vi "Brewer Palette Dialog v2.vi"() -> (0 "OK?":bool, 1 "Cancelled?":bool, 2 "Interpolate?":bool, 3 "Selected Palette Colors":u32[](array[colorbox]), 5 "Palette Name (# Colors)":string)   [LabVIEW 2021]
doc: "The Palette Colors array returned was chosen by the user while it was displayed vertically.\nIn other words, the top color is in fact color index 0, while the bottom color is in fact the last color in the array.\nTo use this array for a color ramp (or color scale), this array will need to be inverted to obtain the same visual effect."
panel:
  in  "Show Tip Strip":bool
  out "Max  # Colors":i32=3 min=3 max=12 step=1
  in  "About":bool
  in  "Interpolate":bool
  in  "Flip Order":bool
  out "Color Ramp":dbl(ramp)
  in  "Palette List":string(combo)
  in  "Cancel":bool
  in  "OK":bool
  out "Palette Colors":u32[](array[colorbox])
  out "# Palettes":i32=3 min=3 max=12 step=1
  in  "Category":T1(ring)
  in  "photocopy safe":bool
  in  "printer friendly":bool
  in  "colorblind safe":bool
  in  "# Colors":i32=3 min=3 max=15 step=1
  in  "Background":u32(colorbox)=16777226
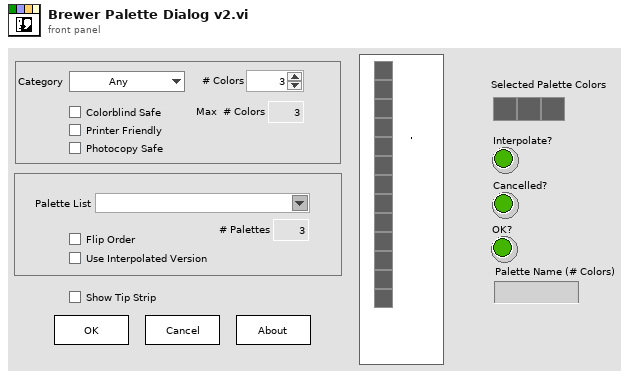
[diagram p1: front panel]
types:
  T1 = enum16{"Any", "Sequential", "Diverging", "Qualitative"}
  T2 = cluster{"Category":enum16{"Any", "Sequential", "Diverging", "Qualitative"}, "photocopy safe":bool, "printer friendly":bool, "colorblind safe":bool, "# Colors":i32, "Flip Order":bool}
  T3 = typedef "Color Brewer Palette.ctl" = cluster{"Color Array":u32[], "Palette Name":string, "Number of Colors":i32, "Palette Category":string, "Color Blind Safe":bool, "Printer Friendly":bool, "Photocopy Safe":bool}
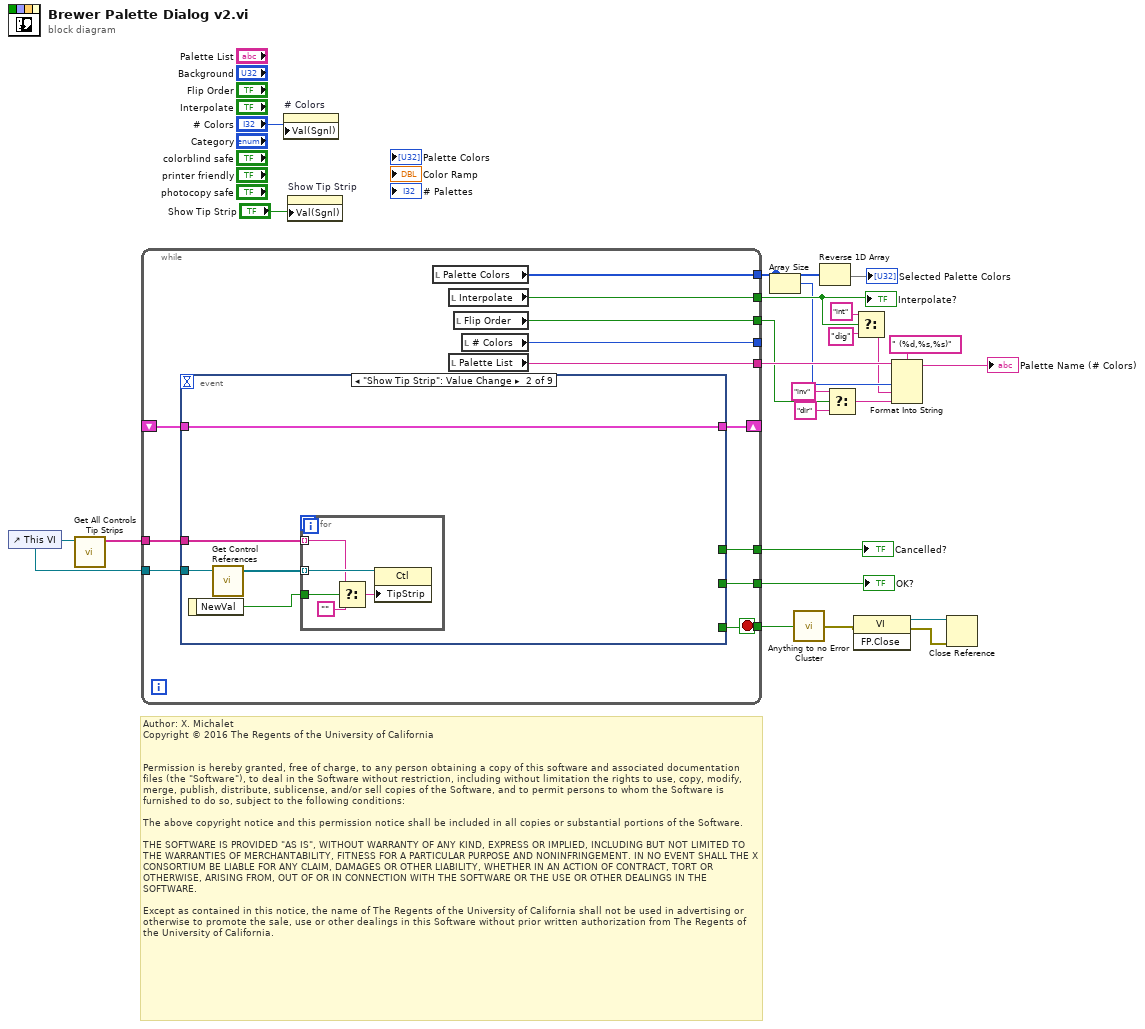
[diagram p0: block diagram]
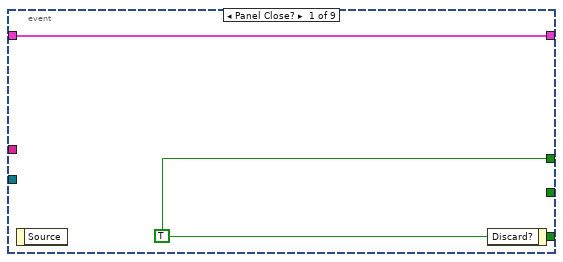
[diagram p2: hidden frame]
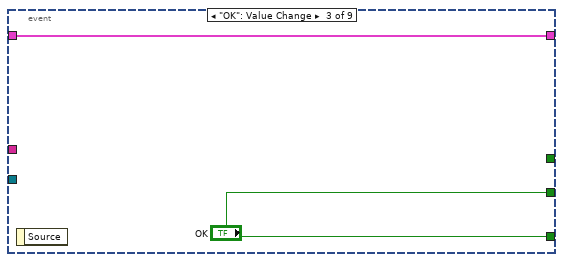
[diagram p3: hidden frame]
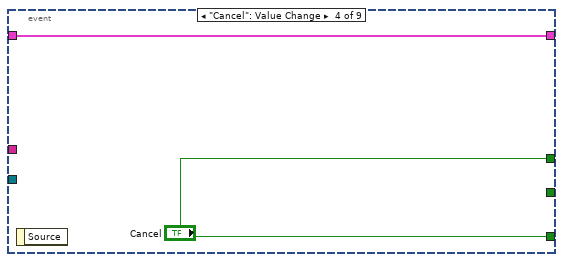
[diagram p4: hidden frame]
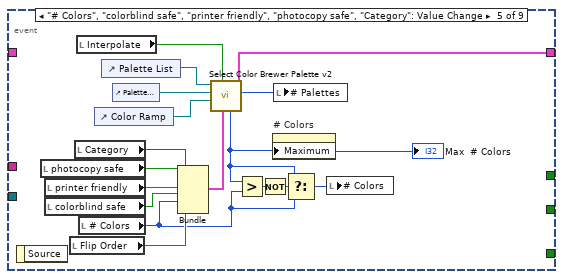
[diagram p5: hidden frame]
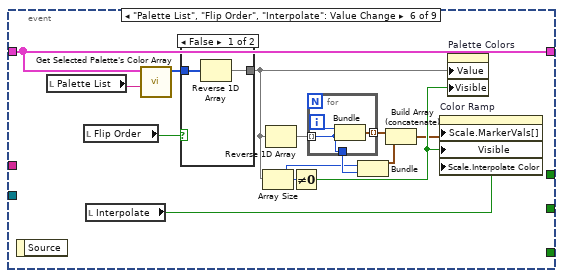
[diagram p6: hidden frame]
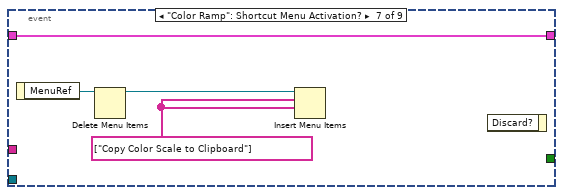
[diagram p8: hidden frame]
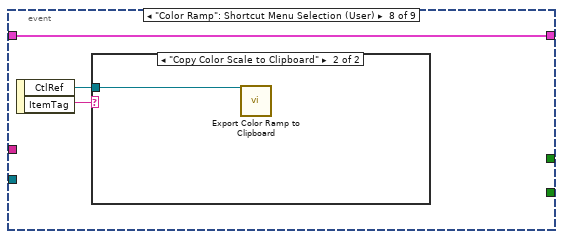
[diagram p9: hidden frame]
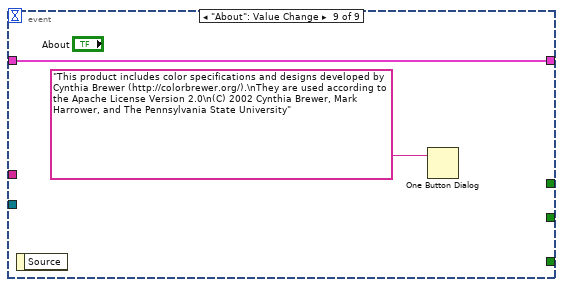
[diagram p11: hidden frame]
diagram:
  # "Author: X. Michalet\nCopyright © 2016 The Regents of the University of California\n \n\nPermission is hereby granted, free of charge, to any person obtaining a copy of this software and associated documentation files (the \"Software\"), to deal in the Software without restriction, including without limitation the rights to use, copy, modify, merge, publish, distribute, sublicense, and/or sell copies of the Software, and to permit persons to whom the Software is furnished to do so, subject to the following conditions:\n\nThe above copyright notice and this permission notice shall be included in all copies or substantial portions of the Software.\n\nTHE SOFTWARE IS PROVIDED \"AS IS\", WITHOUT WARRANTY OF ANY KIND, EXPRESS OR IMPLIED, INCLUDING BUT NOT LIMITED TO THE WARRANTIES OF MERCHANTABILITY, FITNESS FOR A PARTICULAR PURPOSE AND NONINFRINGEMENT. IN NO EVENT SHALL THE X CONSORTIUM BE LIABLE FOR ANY CLAIM, DAMAGES OR OTHER LIABILITY, WHETHER IN AN ACTION OF CONTRACT, TORT OR OTHERWISE, ARISING FROM, OUT OF OR IN CONNECTION WITH THE SOFTWARE OR THE USE OR OTHER DEALINGS IN THE SOFTWARE.\n\nExcept as contained in this notice, the name of The Regents of the University of California shall not be used in advertising or otherwise to promote the sale, use or other dealings in this Software without prior written authorization from The Regents of the University of California."
  n1 = control-ref of="This VI"() -> (w4:refnum<vi>)
  n2 = call "Get All Controls Tip Strips.vi"("VI Ref"=w4) -> ("Controls Tip Strips"=w6:string[])  [unwired: 9 in, 1 out]
  n3 = while {
    shift-right: [w36] -> _
    shift-left: _ -> [w35]
    tunnel: [w34] -> w24
    tunnel: [w33] -> w23
    tunnel: [w32] -> w20
    tunnel: [w31] -> _
    tunnel: [w30] -> w17
    tunnel: [w29] -> w15
    tunnel: [w28] -> w16
    tunnel: w4 -> [w27]
    tunnel: w6 -> [w26]
    tunnel: [w25] -> w2
    stop <- w25 stop-if-true
    n4 = event shown="[1] \"Show Tip Strip\": Value Change" {
      selector: _ -> [_ _ _ _ _ _ _ _ _]
      dyn-events: _ -> [_ _ _ _ _ _ _ _ _]
      timeout: _ -> [_ _ _ _ _ _ _ _ _]
      tunnel: [w37 _ "OK" "Cancel" _ _ _ _ _] -> w25
      tunnel: [w38 w43 w49 w51 w63 w82 w92 w95 w98] -> w36
      tunnel: w35 -> [w38 w43 w49 w51 _ w82 w92 w95 w98]
      tunnel: [_ _ "OK" _ _ _ _ _ _] -> w34
      tunnel: [w37 _ _ "Cancel" _ _ _ _ _] -> w33
      tunnel: w27 -> [_ w42 _ _ _ _ _ _ _]
      tunnel: w26 -> [_ w39 _ _ _ _ _ _ _]
      event Panel Close? {
        w37 = TRUE ("Discard?")
        n5 = event-data() -> ()  [unwired: 1 in, 1 out]
        n6 = event-data("Discard?"=w37) -> ()  [unwired: 1 in, 1 out]
      }
      event "Show Tip Strip": Value Change {
        n7 = event-data() -> ("NewVal"=w40:bool)  [unwired: 1 in]
        n8 = call "Get Control References.vi"("VI  Ref"=w42) -> ("Controls[]"=w41:refnum<vi>[])  [unwired: 2 in, 2 out]
        n9 = for {
          tunnel: w41 -> [w48] mode=indexing
          tunnel: w40 -> [w47]
          tunnel: w39 -> [w45] mode=indexing
          n10 = Select(t=w45, s=w47, f="") -> (s? t:f=w46:string)
          n11 = property class="Ctl"(reference=w48, "TipStrip"=w46) -> ()  [unwired: 1 in, 2 out]
        }
      }
      event "OK": Value Change {
        n12 = event-data() -> ()  [unwired: 1 in, 1 out]
      }
      event "Cancel": Value Change {
        n13 = event-data() -> ()  [unwired: 1 in, 1 out]
      }
      event "# Colors", "colorblind safe", "printer friendly", "photocopy safe", "Category": Value Change {
        n14 = event-data() -> ()  [unwired: 1 in, 1 out]
        n15 = local read "photocopy safe"() -> (w68:bool)
        n16 = local read "printer friendly"() -> (w67:bool)
        n17 = local read "colorblind safe"() -> (w66:bool)
        n18 = local read "Flip Order"() -> (w59:bool)
        n19 = local read "Category"() -> (w69:T1)
        n20 = local read "Interpolate"() -> (w53:bool)
        n21 = local read "# Colors"() -> (w57:i32)
        n22 = control-ref of="Color Ramp"() -> (w60:refnum<vi>)
        n23 = control-ref of="Palette List"() -> (w62:refnum<vi>)
        n24 = control-ref of="Palette Colors"() -> (w65:refnum<vi>)
        n25 = Bundle("Category"=w69, "photocopy safe"=w68, "printer friendly"=w67, "colorblind safe"=w66, "# Colors"=w57, "Flip Order"=w59) -> (w61:T2)  [unwired: 1 in]
        n26 = call "Select Color Brewer Palette v2.vi"("User Choices"=w61, "Interpolate"=w53, "Color Ramp Refnum"=w60, "Palette Colors"=w65, "Palette List Refnum"=w62) -> ("# Palettes"=w64:i32, "Available Palettes"=w63:T3[], "Compatible Max # Colors"=w54:i32)  [unwired: 2 in, 2 out]
        "Max  # Colors" <- w54
        n27 = Greater?(x=w54, y=w57) -> (0:w58:bool)
        n28 = Not(x=w58) -> (.not. x?=w55:bool)
        n29 = property on="# Colors" class="DigNum (strict)"("Maximum"=w54) -> ()  [unwired: 2 in, 2 out]
        n30 = local write "# Palettes"(w64) -> ()
        n31 = Select(t=w54, s=w55, f=w57) -> (s? t:f=w56:i32)
        n32 = local write "# Colors"(w56) -> ()
      }
      event "Palette List", "Flip Order", "Interpolate": Value Change {
        n33 = event-data() -> ()  [unwired: 1 in, 1 out]
        n34 = local read "Palette List"() -> (w77:string)
        n35 = local read "Flip Order"() -> (w81:bool)
        n36 = local read "Interpolate"() -> (w74:bool)
        n37 = call "Get Selected Palette's Color Array.vi"("Selected Palette"=w77, "Palette Specifications"=w82) -> ("Palette Colors"=w80:u32[])  [unwired: 8 in, 1 out]
        n38 = case shown="False" w81 {
          tunnel: w80 -> [w87 w88]
          tunnel: [w86 w88] -> w76
          frame False {
            n39 = Reverse 1D Array(array=w87) -> (reversed array=w86:u32[])
          }
          frame True {
          }
        }
        n40 = Array Size(array=w76) -> (size(s)=w70:i32)
        n41 = Reverse 1D Array(array=w76) -> (reversed array=w79:u32[])
        n42 = Not Equal To 0?(x=w70) -> (x != 0?=w75:bool)
        n43 = for {
          tunnel: w79 -> [w83] mode=indexing
          tunnel: [w84] -> w78 mode=indexing
          tunnel: [w83] -> w71
          i -> [w85]
          n44 = Bundle(w85, "Color Box"=w83) -> (w84:cluster{i32, "Color Box":u32})  [unwired: 1 in]
        }
        n45 = Bundle(w70, "Color Box"=w71) -> (w72:cluster{i32, "Color Box":u32})  [unwired: 1 in]
        n46 = Build Array (concatenate)(w78, w72) -> (w73:cluster{i32, "Color Box":u32}[])
        n47 = property on="Color Ramp" class="ColRmp (strict)"("Scale.MarkerVals[]"=w73, "Visible"=w75, "Scale.Interpolate Color"=w74) -> ()  [unwired: 2 in, 2 out]
        n48 = property on="Palette Colors" class="Arr (strict)"("Value"=w76, "Visible"=w75) -> ()  [unwired: 2 in, 2 out]
      }
      event "Color Ramp": Shortcut Menu Activation? {
        w90 = string[] ["Copy Color Scale to Clipboard"] ("item names")
        n49 = event-data() -> ("MenuRef"=w89:refnum<k9>)  [unwired: 1 in]
        n50 = Delete Menu Items(9:w89) -> (3:w91:refnum<k9>)  [unwired: 3 in, 1 out]
        n51 = Insert Menu Items(7:w90, 8:w90, 9:w91) -> ()  [unwired: 3 in, 3 out]
        n52 = event-data() -> ()  [unwired: 2 in, 1 out]
      }
      event "Color Ramp": Shortcut Menu Selection (User) {
        n53 = event-data() -> ("CtlRef"=w93:refnum<vi>, "ItemTag"=w94:string)  [unwired: 1 in]
        n54 = case shown="\"Copy Color Scale to Clipboard\"" w94 {
          tunnel: w93 -> [_ w96]
          frame "", Default {
          }
          frame "Copy Color Scale to Clipboard" {
            n55 = call "Export Color Ramp to Clipboard.vi"("ColorRamp in"=w96) -> ()  [unwired: 11 in]
          }
        }
      }
      event "About": Value Change {
        n56 = event-data() -> ()  [unwired: 1 in, 1 out]
        n57 = One Button Dialog(message="This product includes color specifications and designs developed by Cynthia Brewer (http://colorbrewer.org/).\nThey are used according to the Apache License Version 2.0\n(C) 2002 Cynthia Brewer, Mark Harrower, and The Pennsylvania State University" ("Text")) -> ()  [unwired: 1 in, 1 out]
      }
    }
    n58 = local read "Palette Colors"() -> (w29:u32[])
    n59 = local read "Interpolate"() -> (w30:bool)
    n60 = local read "Palette List"() -> (w32:string)
    n61 = local read "Flip Order"() -> (w28:bool)
    n62 = local read "# Colors"() -> (w31:i32)
  }
  "OK?" <- w24
  "Cancelled?" <- w23
  "Interpolate?" <- w17
  n63 = property on="# Colors" class="DigNum (strict)"("Val(Sgnl)"="# Colors") -> ()  [unwired: 2 in, 2 out]
  n64 = property on="Show Tip Strip" class="Bool (strict)"("Val(Sgnl)"="Show Tip Strip") -> ()  [unwired: 2 in, 2 out]
  n65 = Array Size(array=w15) -> (size(s)=w14:i32)
  n66 = call "Anything to no Error Cluster.vi"("Variant"=w2) -> ("Error Out"=w1:errorcluster)  [unwired: 8 in]
  n67 = Reverse 1D Array(array=w15) -> (reversed array=→"Selected Palette Colors":u32[])
  n68 = Select(t="inv" ("input 2"), s=w16, f="dir") -> (s? t:f=w8:string)
  n69 = invoke class="VI" method="FP.Close"(error in=w1) -> (reference out=w21:refnum<vi>, error out=w3:errorcluster)  [unwired: 2 in, 1 out]
  n70 = Select(t="int" ("input 2"), s=w17, f="dig") -> (s? t:f=w10:string)
  n71 = Format Into String(format string=" (%d,%s,%s)", initial string=w20, w14, w10, w8) -> (resulting string=→"Palette Name (# Colors)":string)  [unwired: 1 in, 1 out]
  n72 = Close Reference(reference=w21, error in (no error)=w3) -> ()  [unwired: 1 out]
